vi "Update Bind Method Constants.vi"(7 "RPC Method Parameters":T1[](array[typedef]), 8 "error in (no error)":errorcluster, 10 "RPC Method Name":string, 11 "VI in":refnum<vi>) -> (0 "error out":errorcluster, 3 "VI out":refnum<vi>)   [LabVIEW 2019, in "gRPC Scripting Tools.lvlib"]
uses:
  gRPC Scripting Tools.lvlib
  TypeDefs/RPC Method Parameters.ctl
  <vilib>/Utility/traverseref.llb/TRef TravTarget.ctl
  <vilib>/Utility/traverseref.llb/VI Scripting - Traverse.lvlib
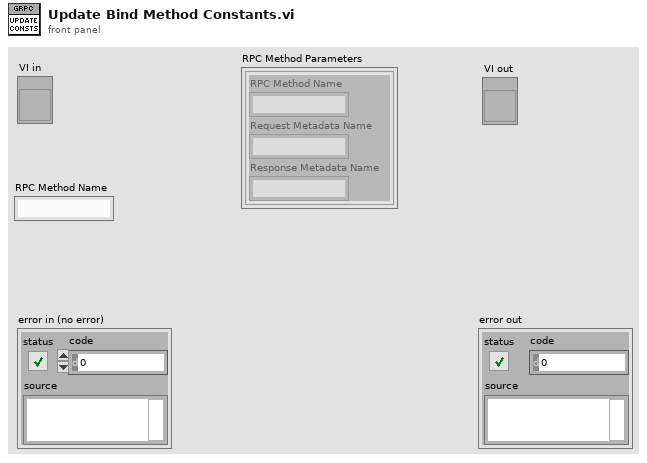
[diagram p1: front panel]
types:
  T1 = typedef "gRPC Scripting Tools.lvlib/RPC Method Parameters.ctl" = cluster{"RPC Method Name":string, "Request Metadata Name":string, "Response Metadata Name":string}
  T2 = typedef "TRef TravTarget.ctl" = enum16{"FP", "BD", "Other"}
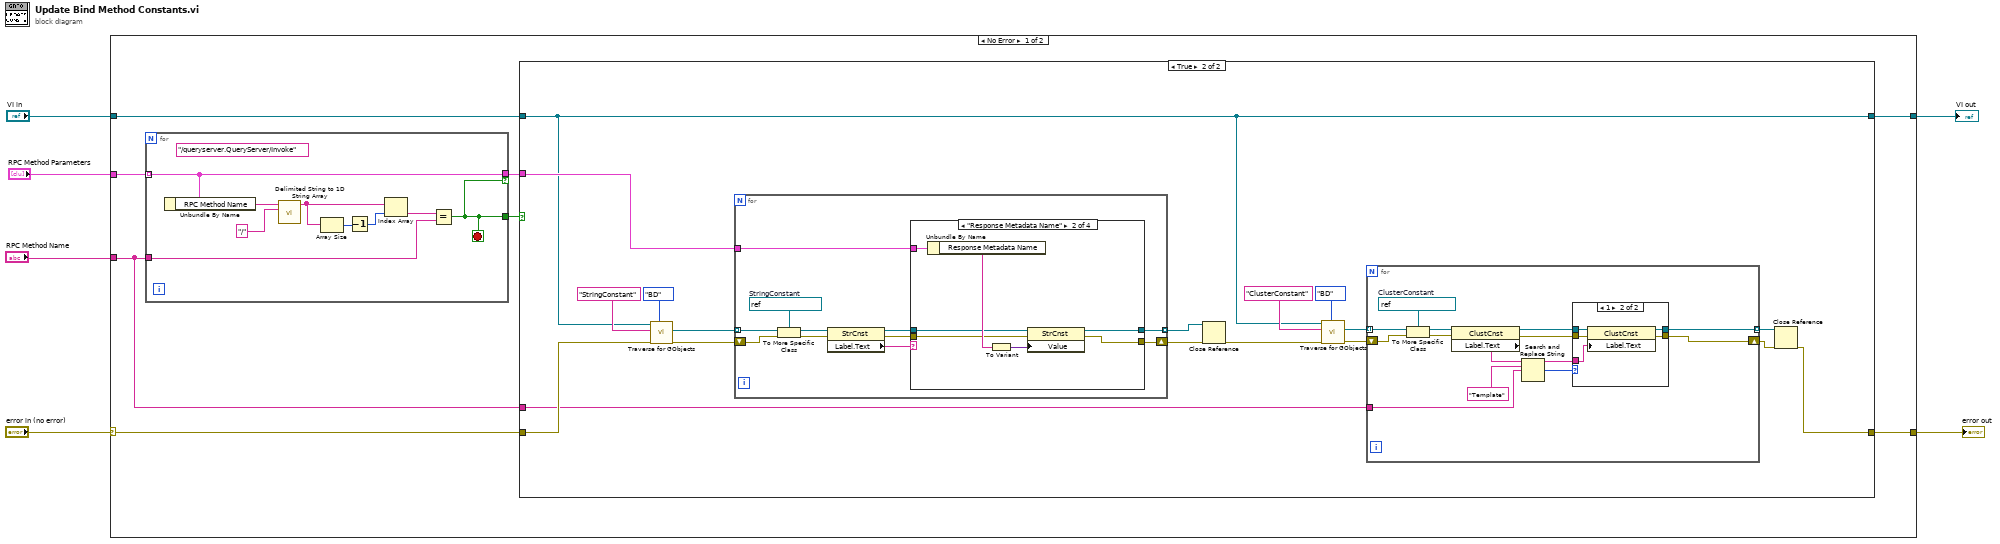
[diagram p0: block diagram]
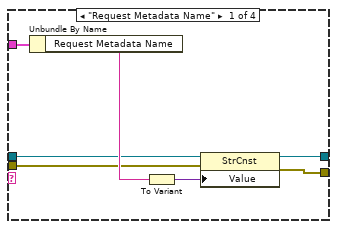
[diagram p4: hidden frame]
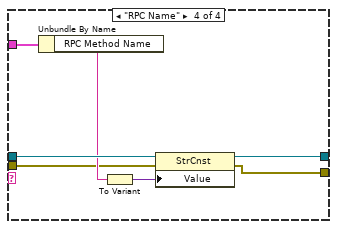
[diagram p6: hidden frame]
diagram:
  n1 = case shown="No Error" "error in (no error)" {
    selector: "error in (no error)" -> [w9 w100]
    tunnel: [w14 w100] -> w6
    tunnel: "VI in" -> [w13 w99]
    tunnel: "RPC Method Parameters" -> [w12 _]
    tunnel: "RPC Method Name" -> [w7 _]
    tunnel: [w8 w99] -> w1
    frame No Error {
      n2 = for {
        tunnel: w12 -> [w91] mode=indexing
        tunnel: w7 -> [w92]
        tunnel: [w91] -> w10 if=w90
        tunnel: [w90] -> w11
        stop <- w90 stop-if-true
        (unwired) "/queryserver.QueryServer/Invoke" ("delimited string")
        n3 = Unbundle By Name(w91) -> ("RPC Method Name"=w97:string)
        n4 = call <vilib>:"Delimited String to 1D String Array.vi"("delimiter"="/", "delimited string"=w97) -> ("string array"=w94:string[])  [unwired: 9 in]
        n5 = Array Size(array=w94) -> (size(s)=w96:i32)
        n6 = Decrement(x=w96) -> (x-1=w95:i32)
        n7 = Index Array(array=w94, index=w95) -> (element=w93:string)
        n8 = Equal?(x=w93, y=w92) -> (x = y?=w90:bool)
      }
      n9 = case shown="True" w11 {
        tunnel: [w16 w18] -> w14
        tunnel: w9 -> [w16 w34]
        tunnel: w13 -> [w15 w23]
        tunnel: w10 -> [_ w30]
        tunnel: [w15 w23] -> w8
        tunnel: w7 -> [_ w20]
        frame False {
          # "#TODO - throw an error as the method is undefined ?"
        }
        frame True {
          n10 = call <vilib>:"Traverse for GObjects.vi"("Traverse Target"=TRef_TravTarget."BD", "error in (no error)"=w34, "Class Name"="StringConstant", "VI Refnum"=w23) -> ("error out"=w31:errorcluster, "References"=w26:refnum<vi>[])  [unwired: 4 in, 2 out]
          n11 = for {
            tunnel: w26 -> [w65] mode=indexing
            shift-right: [w57] -> w27
            shift-left: w31 -> [w64]
            tunnel: w30 -> [w60]
            tunnel: [w56] -> w25 mode=indexing
            w66 = refnum<vi> refnum  # StringConstant
            n12 = To More Specific Class(target class=w66, reference=w65, error in=w64) -> (specific class reference=w63:refnum<vi>, error out=w62:errorcluster)
            n13 = property class="StrCnst"(reference=w63, error in=w62) -> (reference out=w59:refnum<vi>, error out=w58:errorcluster, "Label.Text"=w61:string)
            n14 = case shown="\"Response Metadata Name\"" w61 {
              tunnel: w60 -> [w68 w78 _ w89]
              tunnel: w59 -> [w70 w76 w81 w88]
              tunnel: w58 -> [w71 w77 w82 w85]
              tunnel: [w69 w75 w82 w84] -> w57
              tunnel: [w67 w74 w81 w83] -> w56
              frame "Request Metadata Name" {
                n15 = Unbundle By Name(w68) -> ("Request Metadata Name"=w73:string)
                n16 = To Variant(anything=w73) -> (Variant=w72:variant)
                n17 = property class="StrCnst"(reference=w70, error in=w71, "Value"=w72) -> (reference out=w67:refnum<vi>, error out=w69:errorcluster)
              }
              frame "Response Metadata Name" {
                n18 = Unbundle By Name(w78) -> ("Response Metadata Name"=w80:string)
                n19 = To Variant(anything=w80) -> (Variant=w79:variant)
                n20 = property class="StrCnst"(reference=w76, error in=w77, "Value"=w79) -> (reference out=w74:refnum<vi>, error out=w75:errorcluster)
              }
              frame "None", Default {
              }
              frame "RPC Name" {
                n21 = Unbundle By Name(w89) -> ("RPC Method Name"=w87:string)
                n22 = To Variant(anything=w87) -> (Variant=w86:variant)
                n23 = property class="StrCnst"(reference=w88, error in=w85, "Value"=w86) -> (reference out=w83:refnum<vi>, error out=w84:errorcluster)
              }
            }
          }
          n24 = Close Reference(reference=w25, error in (no error)=w27) -> (error out=w24:errorcluster)
          n25 = call <vilib>:"Traverse for GObjects.vi"("Traverse Target"=TRef_TravTarget."BD", "error in (no error)"=w24, "Class Name"="ClusterConstant", "VI Refnum"=w23) -> ("error out"=w22:errorcluster, "References"=w21:refnum<vi>[])  [unwired: 4 in, 2 out]
          n26 = for {
            tunnel: w21 -> [w47] mode=indexing
            shift-right: [w36] -> w19
            shift-left: w22 -> [w46]
            tunnel: w20 -> [w41]
            tunnel: [w35] -> w17 mode=indexing
            w48 = refnum<vi> refnum  # ClusterConstant
            n27 = To More Specific Class(target class=w48, reference=w47, error in=w46) -> (specific class reference=w45:refnum<vi>, error out=w44:errorcluster)
            n28 = property class="ClustCnst"(reference=w45, error in=w44) -> (reference out=w40:refnum<vi>, error out=w39:errorcluster, "Label.Text"=w42:string)
            n29 = Search and Replace String(input string=w42, search string="Template", replace string=w41) -> (result string=w37:string, number of replacements=w38:i32)  [unwired: 5 in, 2 out]
            n30 = case shown="1" w38 {
              tunnel: w40 -> [w50 w55]
              tunnel: [w50 w54] -> w35
              tunnel: [w49 w53] -> w36
              tunnel: w39 -> [w49 w52]
              tunnel: w37 -> [_ w51]
              frame 0, Default {
              }
              frame 1 {
                n31 = property class="ClustCnst"(reference=w55, error in=w52, "Label.Text"=w51) -> (reference out=w54:refnum<vi>, error out=w53:errorcluster)
              }
            }
          }
          n32 = Close Reference(reference=w17, error in (no error)=w19) -> (error out=w18:errorcluster)
        }
      }
    }
    frame Error {
    }
  }
  "error out" <- w6
  "VI out" <- w1
